vi "Event Nested Teardown.vi"(11 "jettl Queue Actor in":refnum<class "jettl Queue Actor.lvclass">) -> (3 "jettl Queue Actor out":refnum<class "jettl Queue Actor.lvclass">)   [LabVIEW 2021, in "jettl.lvlib" / "jettl Queue Actor.lvclass"]
uses:
  jettl Queue Actor.lvclass
  Actor/Msgs/Teardown/Teardown Msg/Teardown Msg.lvclass
  C:/git/jettl/src/Actor/Msg/Msg.lvclass
  jettl Queue Actor.lvclass/jettl Queue Actor.ctl
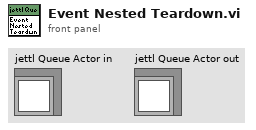
[diagram p1: front panel]
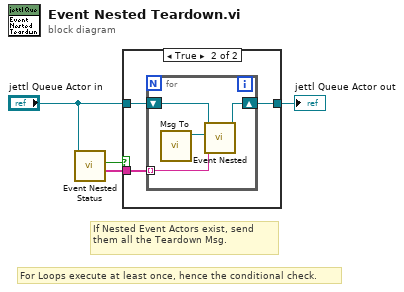
[diagram p0: block diagram]
diagram:
  # "If Nested Event Actors exist, send them all the Teardown Msg."
  # "For Loops execute at least once, hence the conditional check."
  n1 = call-dynamic "Event Nested Status.vi"("jettl Queue Actor in"="jettl Queue Actor in") -> ("Event Nested Aliases"=w3:string[], "Any Exist?"=w4:bool)  [unwired: 8 in, 1 out]
  n2 = case shown="True" w4 {
    tunnel: [w5 w8] -> w1
    tunnel: "jettl Queue Actor in" -> [w5 w7]
    tunnel: w3 -> [_ w6]
    frame False {
    }
    frame True {
      n3 = for {
        tunnel: w6 -> [w9] mode=indexing
        shift-right: [w11] -> w8
        shift-left: w7 -> [w12]
        n4 = call "Msg To.vi"() -> ("Teardown Msg out"=w10:refnum<class "Teardown Msg.lvclass">)  [unwired: 11 in]
        n5 = call-dynamic "Event Nested.vi"("Alias"=w9, "Msg"=w10, "jettl Queue Actor in"=w12) -> ("jettl Queue Actor out"=w11:refnum<class "jettl Queue Actor.lvclass">)  [unwired: 8 in]
      }
    }
  }
  "jettl Queue Actor out" <- w1
